vi "SLSC Write CS Bits.vi"(10 "CS Bit Value/Slot #":u8, 11 "CS Bits":T1={"CS Bit 1"="Connector0/DIO0", "CS Bit 2"="Connector0/DIO0", "CS Bit 3"="Connector0/DIO0", "CS Bit 4"="Connector0/DIO0"}) -> ()   [LabVIEW 2014, in "SLSC FPGA Toolkit.lvlib"]
uses:
  SLSC FPGA Toolkit.lvlib
  Source/Shared/SPI Utility/CS Bits.ctl
  <vilib>/rvi/eio/common/nirviEmuTemplateMethod_errors.vi
  <vilib>/eio/EIONode/EIONode.xnode
  Source/Shared/SLSC configuration Shared.lvlib
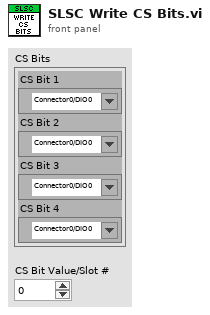
[diagram p1: front panel]
types:
  T1 = typedef "SLSC configuration Shared.lvlib/CS Bits.ctl" = cluster{"CS Bit 1":refnum<k21>, "CS Bit 2":refnum<k21>, "CS Bit 3":refnum<k21>, "CS Bit 4":refnum<k21>}
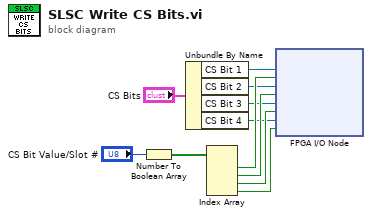
[diagram p0: block diagram]
diagram:
  n1 = Number To Boolean Array(number="CS Bit Value/Slot #") -> (Boolean array=w6:bool[])
  n2 = Unbundle By Name("CS Bits") -> ("CS Bit 1"=w1:refnum<k21>, "CS Bit 2"=w2:refnum<k21>, "CS Bit 3"=w3:refnum<k21>, "CS Bit 4"=w4:refnum<k21>)
  n3 = Index Array(array=w6) -> (element #1=w7:bool, element #2=w8:bool, element #3=w9:bool, element #4=w10:bool)  [unwired: 4 in]
  n4 = xnode "FPGA I/O Node"("I/O Item"=w7, "FPGA I/O In"=w1, "I/O Item"=w8, "FPGA I/O In"=w2, "I/O Item"=w9, "FPGA I/O In"=w3, "I/O Item"=w10, "FPGA I/O In"=w4) -> ()  [unwired: 4 out]
